vi "arreglobidi3.vi"() -> ()   [LabVIEW 2011]
uses:
  arreglobidi3.ctl
panel:
  out "Array":dbl[][](array[numeric])
  # "se deera de ingresar datos en todas las lineas y columnas dejando la ultima columna \nreservada para la suma de  cada una de las lineas y guardando la suma en la ultima columna."
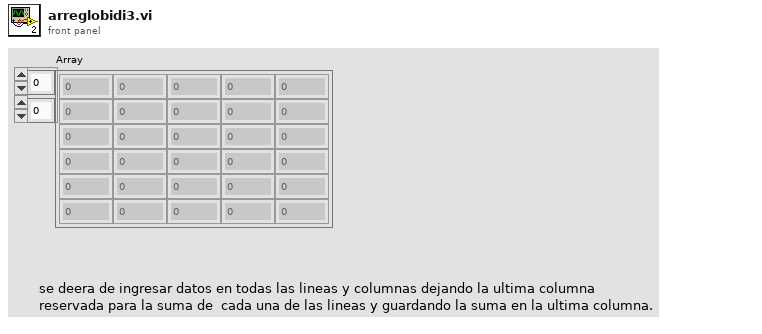
[diagram p1: front panel]
types:
  T1 = typedef "arreglobidi3.ctl" = enum16{"inicializar arreglo", "rellenar arreglo", "sumar lineas", "finalizar"}
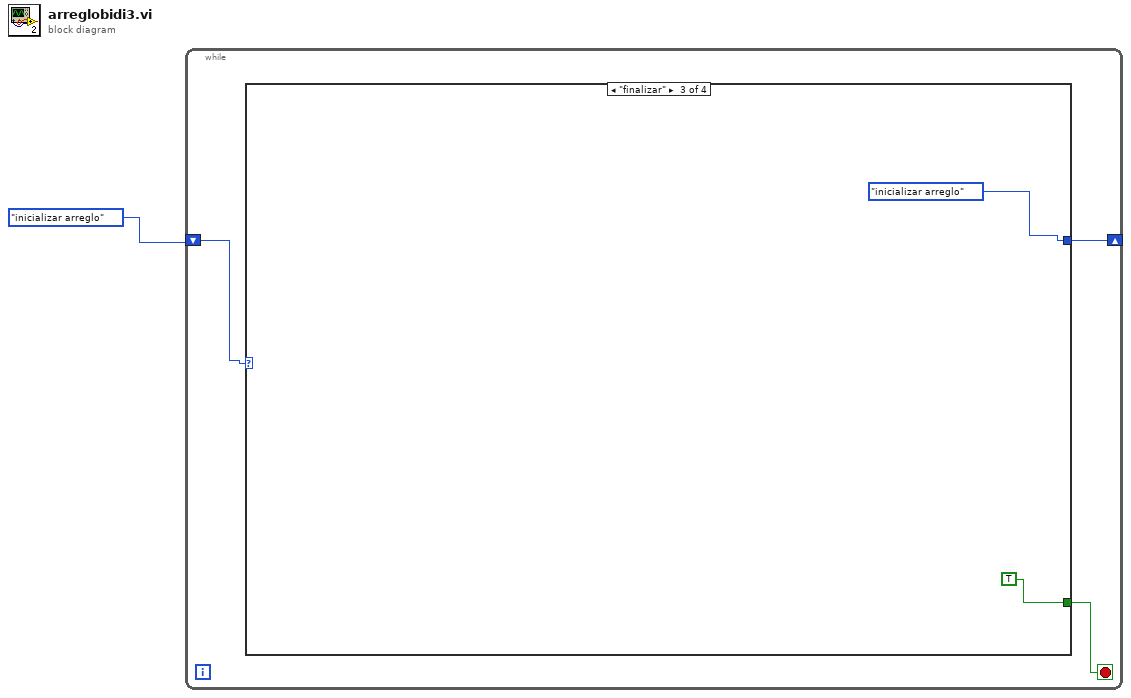
[diagram p0: block diagram]
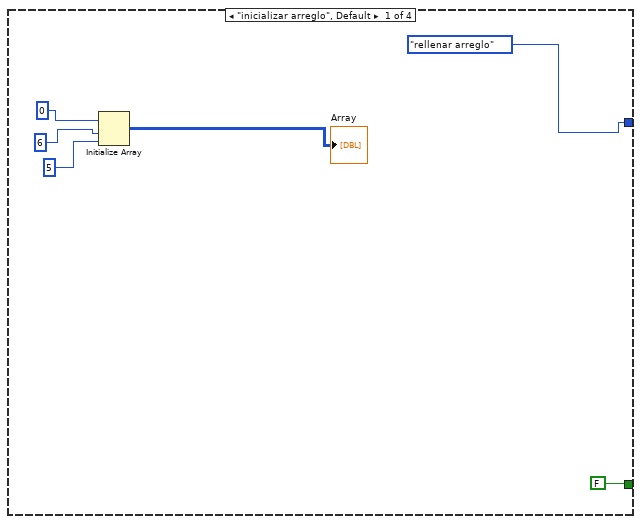
[diagram p2: hidden frame]
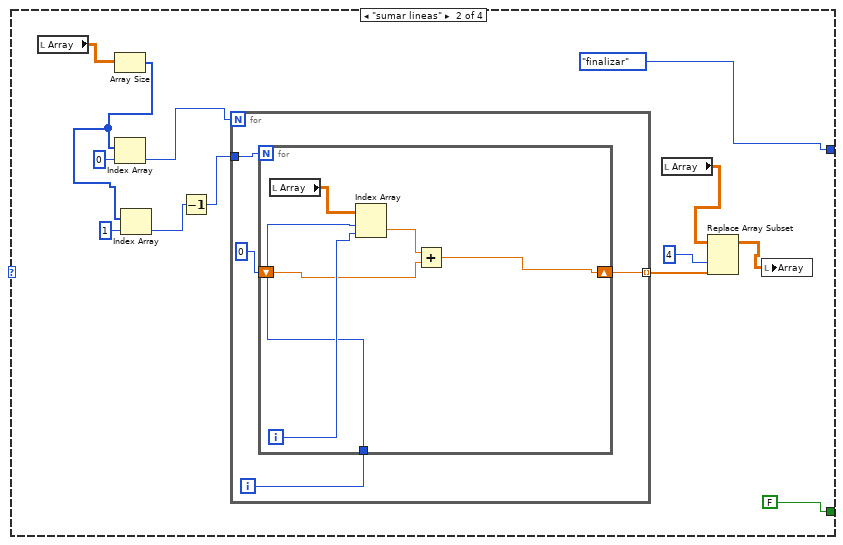
[diagram p3: hidden frame]
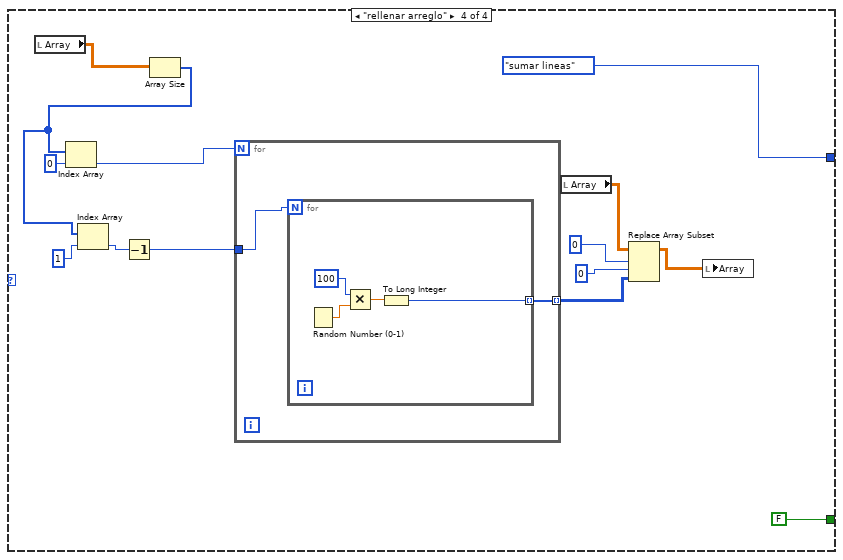
[diagram p4: hidden frame]
diagram:
  n1 = while {
    shift-right: [w3] -> _
    shift-left: arreglobidi3."inicializar arreglo" -> [w4]
    stop <- w2 stop-if-true
    n2 = case shown="\"finalizar\"" w4 {
      tunnel: [arreglobidi3."rellenar arreglo" arreglobidi3."finalizar" arreglobidi3."inicializar arreglo" arreglobidi3."sumar lineas"] -> w3
      tunnel: [FALSE FALSE TRUE FALSE] -> w2
      frame "inicializar arreglo", Default {
        n3 = Initialize Array "Initialize Array"(0, 6, 5) -> (→"Array":i32[][])
      }
      frame "sumar lineas" {
        n4 = local read "Array"() -> (w22:dbl[][])
        n5 = Array Size(array=w22) -> (size(s)=w18:i32[])
        n6 = Index Array(array=w18, index=0) -> (element=w20:i32)
        n7 = Index Array(array=w18, index=1) -> (element=w17:i32)
        n8 = Decrement(x=w17) -> (x-1=w16:i32)
        n9 = for {
          N: w20 -> [_]
          tunnel: w16 -> [w27]
          tunnel: [w24] -> w13 mode=indexing
          i -> [w26]
          n10 = for {
            N: w27 -> [_]
            tunnel: w26 -> [w31]
            shift-right: [w28] -> w24
            shift-left: 0 ("index") -> [w29]
            i -> [w32]
            n11 = local read "Array"() -> (w33:dbl[][])
            n12 = Index Array(array=w33, index (row)=w31, index (col)=w32) -> (element=w30:dbl)
            n13 = Add(x=w30, y=w29) -> (x+y=w28:dbl)
          }
        }
        n14 = local read "Array"() -> (w15:dbl[][])
        n15 = Replace Array Subset "Replace Array Subset"(array=w15, new element=w13, index (col)=4 ("disabled index (col)")) -> (w14:dbl[][])  [unwired: 1 in]
        n16 = local write "Array"(w14) -> ()
      }
      frame "finalizar" {
      }
      frame "rellenar arreglo" {
        n17 = local read "Array"() -> (w47:dbl[][])
        n18 = Array Size(array=w47) -> (size(s)=w43:i32[])
        n19 = Index Array "Index Array"(array=w43, index=0) -> (element=w45:i32)
        n20 = Index Array "Index Array"(array=w43, index=1) -> (element=w42:i32)
        n21 = Decrement(x=w42) -> (x-1=w41:i32)
        n22 = for {
          N: w45 -> [_]
          tunnel: w41 -> [w51]
          tunnel: [w50] -> w38 mode=indexing
          n23 = for {
            N: w51 -> [_]
            tunnel: [w52] -> w50 mode=indexing
            n24 = Random Number (0-1)() -> (number: 0 to 1=w55:dbl)
            n25 = Multiply(x=100, y=w55) -> (x*y=w53:dbl)
            n26 = To Long Integer(number=w53) -> (32bit integer=w52:i32)
          }
        }
        n27 = local read "Array"() -> (w39:dbl[][])
        n28 = Replace Array Subset "Replace Array Subset"(array=w39, new element=w38, index (row)=0, index (col)=0 ("index (row)")) -> (w40:dbl[][])
        n29 = local write "Array"(w40) -> ()
      }
    }
  }
